vi "Aerotech set home.vi"(8 "error in (no error)":errorcluster, 10 "Parsed CMD":T1, 11 "AerotechStage in":refnum<class "AerotechStage.lvclass">) -> (0 "error out":errorcluster, 2 "new commands":string, 3 "AerotechStage out":refnum<class "AerotechStage.lvclass">)   [LabVIEW 2013, in "AerotechStage.lvclass"]
uses:
  AerotechStage.lvclass
  shared/parsed device cmd.ctl
  shared/OnOffTypeDef.ctl
  AerotechStage.lvclass/AerotechStage.ctl
  shared/CompressAndUpdate(Poly)/CompressAndUpdate(Enum).vi
  HomeSingle.vi
  1WireSystem/1WireSystem.lvclass
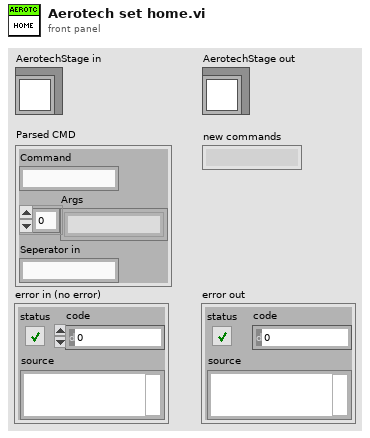
[diagram p1: front panel]
types:
  T1 = typedef "parsed device cmd.ctl" = cluster{"Command":string, "Args":string[], "Seperator in":string}
  T2 = typedef "OnOffTypeDef.ctl" = enum16{"off", "on"}
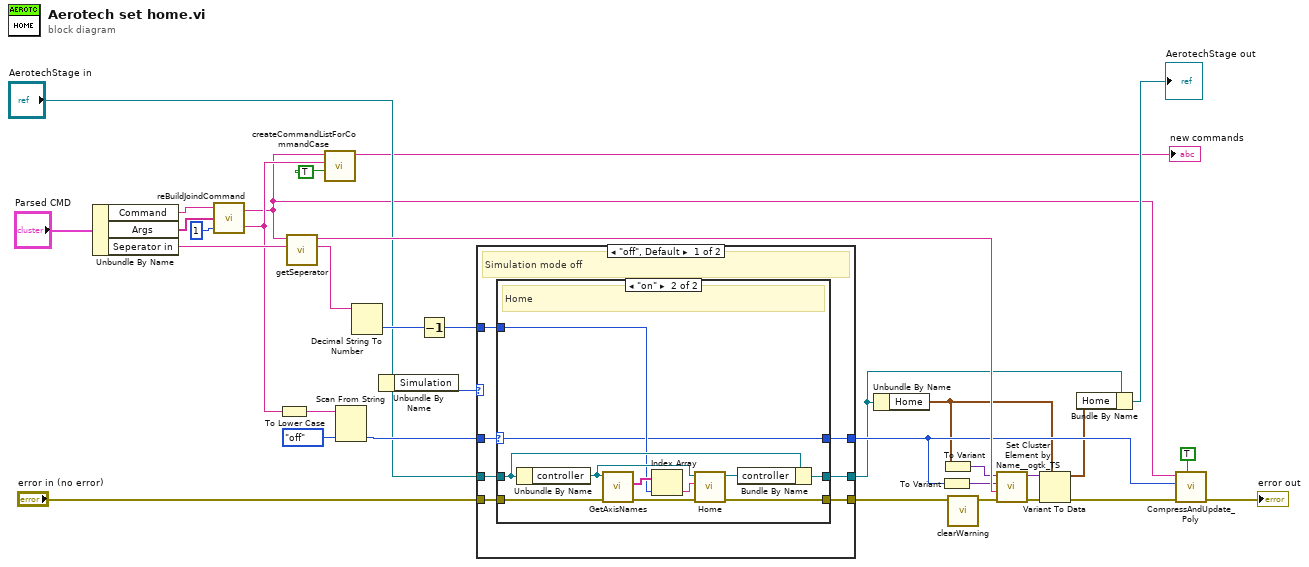
[diagram p0: block diagram]
diagram:
  n1 = Unbundle By Name("Parsed CMD") -> ("Command"=w33:string, "Args"=w31:string[], "Seperator in"=w32:string)
  n2 = call "reBuildJoindCommand.vi"("number of group elements (0)"=1, "Args"=w31, "Command 2"=w33) -> ("Arg"=w10:string, "Command"=w4:string)
  n3 = To Lower Case(string=w10) -> (all lower case string=w9:string)
  n4 = call "getSeperator.vi"("Channel Seperator (\"\")"=w32, "Command"=w4) -> ("Channel"=w16:string, "Seperator (e.g. \"Channel1\")"=w29:string)  [unwired: 8 in]
  n5 = call "createCommandListForCommandCase.vi"("immediate Check (only once)"=TRUE, "setvalue"=w10, "command"=w4) -> ("new commands"=→"new commands":string)  [unwired: 8 in]
  n6 = Scan From String(input string=w9, default 1=OnOffTypeDef."off" ("Settings.Enable.Axis 1")) -> (output 1=w12:T2)  [unwired: 3 in, 3 out]
  n7 = Decimal String To Number(string=w16) -> (number=w14:i32)  [unwired: 2 in, 1 out]
  n8 = Unbundle By Name("AerotechStage in") -> ("Simulation"=w8:T2)
  n9 = Decrement(x=w14) -> (x-1=w15:i32)
  n10 = case shown="\"off\", Default" w8 {
    tunnel: "AerotechStage in" -> [w40 w57]
    tunnel: "error in (no error)" -> [w38 w56]
    tunnel: [w37 w56] -> w25
    tunnel: [w39 w57] -> w24
    tunnel: w12 -> [w36 w55]
    tunnel: w15 -> [w35 _]
    tunnel: [w34 w55] -> w26
    frame "off", Default {
      # "Simulation mode off"
      n11 = case shown="\"on\"" w36 {
        selector: w36 -> [w41 w44]
        tunnel: w40 -> [w42 w54]
        tunnel: [w42 w53] -> w39
        tunnel: w38 -> [w43 w49]
        tunnel: [w43 w52] -> w37
        tunnel: w35 -> [_ w47]
        tunnel: [w41 w44] -> w34
        frame "off", Default {
          # "Disable Axis"
        }
        frame "on" {
          # "Home"
          n12 = Unbundle By Name(w54) -> ("controller"=w50:refnum<k24>)
          n13 = call "GetAxisNames.vi"("error in (no error)"=w49, "controller in"=w50) -> ("error out"=w45:errorcluster, "axis names"=w48:string[])  [unwired: 7 in, 1 out]
          n14 = Index Array(array=w48, index=w47) -> (element=w46:string)
          n15 = call-poly "Home.vi"("error in (no error)"=w45, "axis name"=w46, "controller in"=w50) -> ("error out"=w52:errorcluster, "controller out"=w51:refnum<k24>)  [unwired: 7 in]
          n16 = Bundle By Name(cluster=w54, "controller"=w51) -> (w53:refnum<class "AerotechStage.lvclass">)
        }
      }
    }
    frame "on" {
      # "Simulation mode on"
    }
  }
  n17 = Unbundle By Name(w24) -> ("Home"=w19:cluster{"Axis1":T2, "Axis2":T2, "Axis3":T2})
  n18 = To Variant(anything=w26) -> (Variant=w21:variant)
  n19 = To Variant(anything=w19) -> (Variant=w22:variant)
  n20 = call "clearWarning.vi"("error in (no error)"=w25) -> ("error out"=w23:errorcluster)  [unwired: 10 in]
  n21 = call "Set Cluster Element by Name__ogtk_TS.vi"("error in (no error)"=w23, "Element Name (\"\": New Element Data Name)"=w29, "New Element Value"=w21, "Cluster"=w22) -> ("error out"=w17:errorcluster, "VCluster out"=w18:variant)  [unwired: 5 in, 1 out]
  n22 = Variant To Data(error in=w17, type=w19, Variant=w18) -> (data=w20:cluster{"Axis1":T2, "Axis2":T2, "Axis3":T2}, error out=w27:errorcluster)
  n23 = Bundle By Name(cluster=w24, "Home"=w20) -> (→"AerotechStage out":refnum<class "AerotechStage.lvclass">)
  n24 = call-poly "CompressAndUpdate_Poly.vi"("force CVT update (false)"=TRUE, "error in"=w27, "enum variant"=w26, "command or variable name"=w4) -> ("error out"=→"error out":errorcluster)  [unwired: 7 in]
